vi "CreatePrivateEvents.vi"(8 "error in (no error)":errorcluster, 11 "EmbeddedSMO":refnum<class "Embedded UI.lvclass">) -> (0 "error out":errorcluster, 3 "EmbeddedSMO out":refnum<class "Embedded UI.lvclass">)   [LabVIEW 2019, in "Embedded UI.lvclass"]
doc: "---------------------------------------------------------------\nJKI State Machine Objects™\nhttp://jki.net/state-machine-objects/\nCopyright (C) 2005-2015, JKI <info@jki.net>\nALL RIGHTS RESERVEDJKI State Machine Objects (SMO) 1.0.0.4\nJKI - JKI\nCopyright (c) 2015, JKI"
uses:
  Embedded UI.lvclass
  Typedefs/PrivateEvents--Embedded UI.Get UI State.ctl
  Typedefs/GetUIStateNotifier.ctl
  Typedefs/UI State.ctl
  Typedefs/PrivateEvents--Embedded UI.SetUIState.ctl
  Typedefs/PrivateEvents--Embedded UI.GetSubPanelReference.ctl
  Typedefs/PrivateEvents--Embedded UI.SetSubpanelReference.ctl
  Typedefs/PrivateEvents--Embedded UI.WriteName.ctl
  Typedefs/PrivateEvents--Embedded UI.GetName.ctl
  Embedded UI.lvclass/Embedded UI.ctl
  <vilib>/JKI/JKI SMO/SMO.UI/SMO.UI.lvclass
panel:
  # "For instructions on how to use the JKI State Machine Objects, examples and video tutorials, visit:\nhttp://jki.net/state-machine-objects/\n\nJKI State Machine Objects™\nhttp://jki.net/state-machine-objects/\nCopyright (C) 2005-2015, JKI <info@jki.net>\nALL RIGHTS RESERVED"
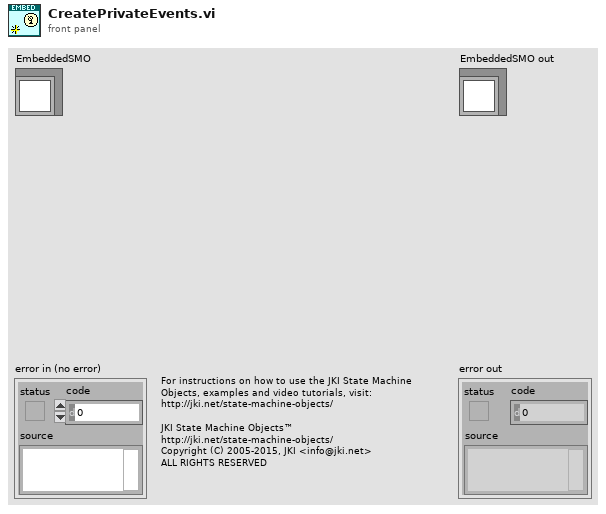
[diagram p1: front panel]
types:
  T1 = typedef "Embedded UI.lvclass/PrivateEvents--Embedded UI.GetName.ctl" = refnum<notifier>
  T2 = typedef "Embedded UI.lvclass/PrivateEvents--Embedded UI.WriteName.ctl" = string
  T3 = typedef "Embedded UI.lvclass/PrivateEvents--Embedded UI.SetSubpanelReference.ctl" = refnum<vi>
  T4 = typedef "Embedded UI.lvclass/PrivateEvents--Embedded UI.GetSubPanelReference.ctl" = refnum<notifier>
  T5 = typedef "Embedded UI.lvclass/PrivateEvents--Embedded UI.SetUIState.ctl" = cluster{"UI State":T6}
  T6 = typedef "Embedded UI.lvclass/UI State.ctl" = enum16{"unknown", "Opened", "Embedded", "Closed"}
  T7 = typedef "Embedded UI.lvclass/PrivateEvents--Embedded UI.Get UI State.ctl" = cluster{"Notifier":T8}
  T8 = typedef "Embedded UI.lvclass/GetUIStateNotifier.ctl" = refnum<notifier>
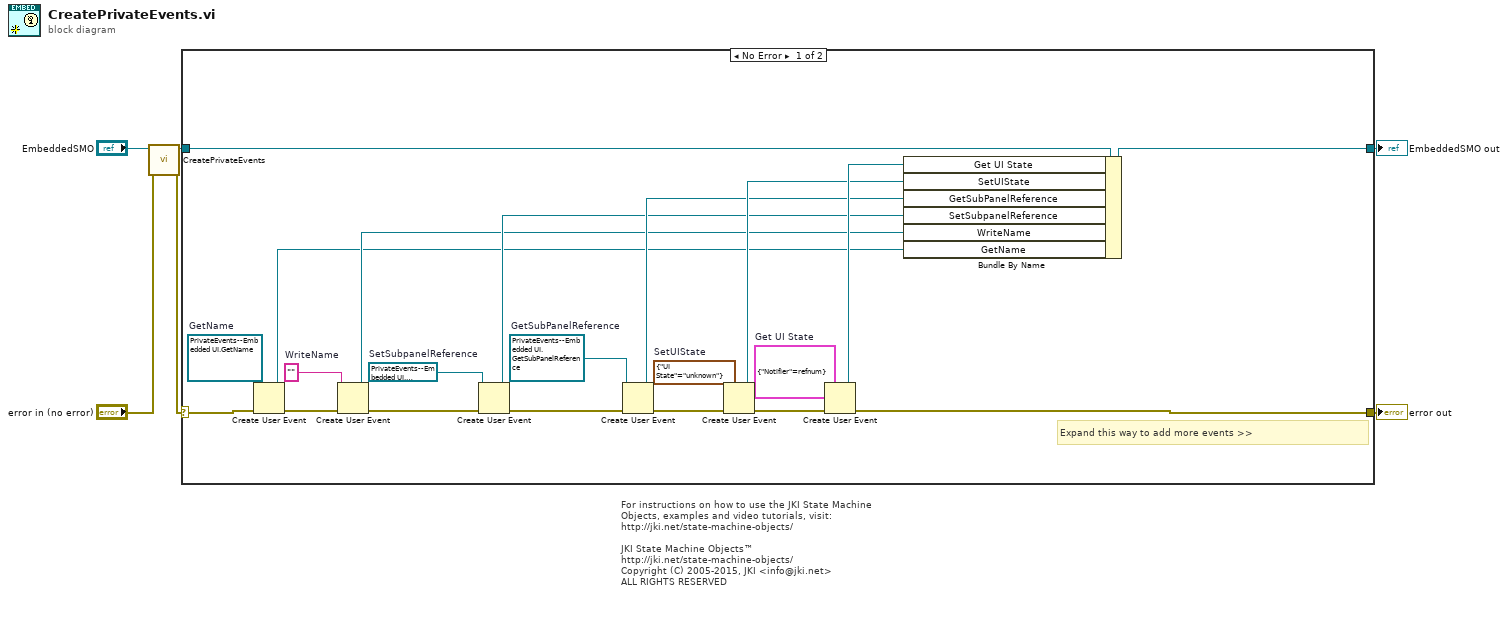
[diagram p0: block diagram]
diagram:
  # "For instructions on how to use the JKI State Machine Objects, examples and video tutorials, visit:\nhttp://jki.net/state-machine-objects/\n\nJKI State Machine Objects™\nhttp://jki.net/state-machine-objects/\nCopyright (C) 2005-2015, JKI <info@jki.net>\nALL RIGHTS RESERVED"
  n1 = call-parent "CreatePrivateEvents.vi"("error in (no error)"="error in (no error)", "SMO.UI"="EmbeddedSMO") -> ("error out"=w1:errorcluster, "SMO.UI out"=w3:refnum<class "Embedded UI.lvclass">)  [unwired: 8 in]
  n2 = case shown="No Error" w1 {
    selector: w1 -> [w26 w29]
    tunnel: [w24 w29] -> w5
    tunnel: [w25 w28] -> w6
    tunnel: w3 -> [w27 w28]
    frame No Error {
      w8 = T1 refnum  # GetName
      w11 = T2 ""  # WriteName
      w14 = T3 refnum  # SetSubpanelReference
      w17 = T4 refnum  # GetSubPanelReference
      w20 = T5 {"UI State"=enum."unknown"}  # SetUIState
      w23 = T7 {"Notifier"=refnum}  # Get UI State
      # "Expand this way to add more events >>"
      n3 = Create User Event(user event datatype=w8, error in=w26) -> (user event=w7:refnum<user-event>, error out=w9:errorcluster)
      n4 = Create User Event(user event datatype=w11, error in=w9) -> (user event=w10:refnum<user-event>, error out=w12:errorcluster)
      n5 = Create User Event(user event datatype=w14, error in=w12) -> (user event=w13:refnum<user-event>, error out=w15:errorcluster)
      n6 = Create User Event(user event datatype=w17, error in=w15) -> (user event=w16:refnum<user-event>, error out=w18:errorcluster)
      n7 = Create User Event(user event datatype=w20, error in=w18) -> (user event=w19:refnum<user-event>, error out=w21:errorcluster)
      n8 = Create User Event(user event datatype=w23, error in=w21) -> (user event=w22:refnum<user-event>, error out=w24:errorcluster)
      n9 = Bundle By Name(cluster=w27, "Get UI State"=w22, "SetUIState"=w19, "GetSubPanelReference"=w16, "SetSubpanelReference"=w13, "WriteName"=w10, "GetName"=w7) -> (w25:refnum<class "Embedded UI.lvclass">)
    }
    frame Error {
    }
  }
  "error out" <- w5
  "EmbeddedSMO out" <- w6
